vi "Filter Log Packet.vi"(10 "Log Packet":T1, 11 "Event Keyword Filter in":refnum<class "Event Keyword Filter.lvclass">) -> (2 "Log?":bool, 3 "Event Keyword Filter out":refnum<class "Event Keyword Filter.lvclass">)   [LabVIEW 2020, in "MVA Framework.lvlib" / "Event Keyword Filter.lvclass"]
uses:
  Event Keyword Filter.lvclass
  Composed Log/Types/Log Packet.ctl
  Composed Log/Types/Log Level.ctl
  Event Keyword Filter.lvclass/Event Keyword Filter.ctl
  Composed Log/Composed Log.lvlib
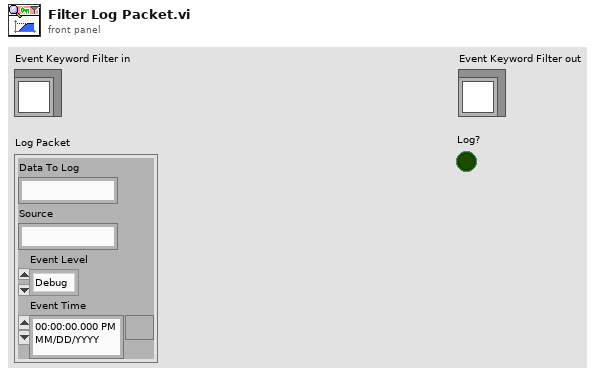
[diagram p1: front panel]
types:
  T1 = typedef "MVA Framework.lvlib/Composed Log.lvlib/Log Packet.ctl" = cluster{"Data To Log":string, "Source":string, "Event Level":T2, "Event Time":timestamp}
  T2 = typedef "MVA Framework.lvlib/Composed Log.lvlib/Log Level.ctl" = enum16{"Debug", "Info", "Warning", "Error", "Critical"}
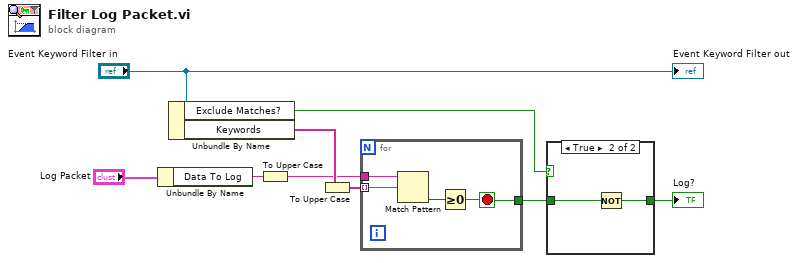
[diagram p0: block diagram]
diagram:
  n1 = Unbundle By Name("Log Packet") -> ("Data To Log"=w6:string)
  n2 = Unbundle By Name("Event Keyword Filter in") -> ("Exclude Matches?"=w1:bool, "Keywords"=w7:string[])
  n3 = To Upper Case(1:w6) -> (0:w5:string)
  n4 = To Upper Case(1:w7) -> (0:w4:string[])
  n5 = for {
    tunnel: w4 -> [w12] mode=indexing
    tunnel: w5 -> [w13]
    tunnel: [w10] -> w2
    stop <- w10 stop-if-true
    n6 = Match Pattern(string=w13, regular expression=w12) -> (offset past match=w11:i32)  [unwired: 1 in, 3 out]
    n7 = Greater Or Equal To 0?(x=w11) -> (x >= 0?=w10:bool)
  }
  n8 = case shown="True" w1 {
    tunnel: [w14 w16] -> w3
    tunnel: w2 -> [w14 w15]
    frame False {
    }
    frame True {
      n9 = Not(x=w15) -> (.not. x?=w16:bool)
    }
  }
  "Log?" <- w3
  "Event Keyword Filter out" <- "Event Keyword Filter in"
